vi "mcs_command_line.vi"() -> ()   [LabVIEW 2013]
panel:
  out "Response":string
  in  "Command":string
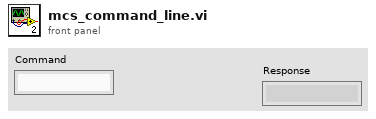
[diagram p1: front panel]
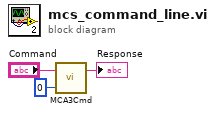
[diagram p0: block diagram]
diagram:
  n1 = call <userlib>:"MCA3Cmd.vi"("MCA #"=0, "Command"="Command") -> ("Response"=→"Response":string)  [unwired: 1 in]
